vi "PrtSc + Crop image.vi"(11 "error in (no error)":errorcluster) -> (0 "error out":errorcluster, 3 "Image Dst Out":T1)   [LabVIEW 2011]
uses:
  <vilib>/vision/Image Controls.llb/IMAQ Image.ctl
  user32.dll
  <vilib>/vision/NI_Vision_Development_Module.lvlib
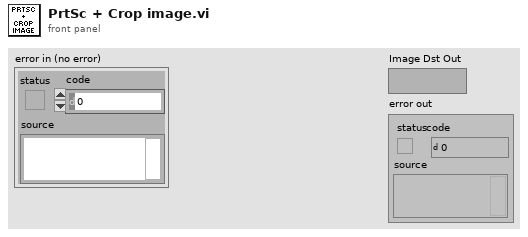
[diagram p1: front panel]
types:
  T1 = typedef "IMAQ Image.ctl" = refnum<image>
  T2 = typedef "Image Type" = u32
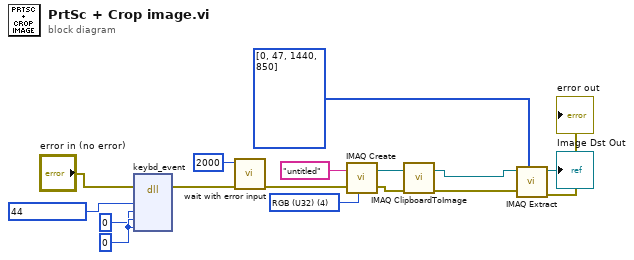
[diagram p0: block diagram]
diagram:
  w8 = T2 4 items=["Grayscale (U8)", "Grayscale (I16)", "Grayscale (SGL)", "Complex (CSG)", "RGB (U32)", "HSL (U32)", "RGB (U64)", "Grayscale (U16)"] ("Image Type")
  w16 = 0
  n1 = dll-call lib="user32.dll" fn="keybd_event"(error in="error in (no error)", u8 44 ("Virtual Key"), i8 0, w16, w16) -> (error out=w11:errorcluster)  [unwired: 7 in, 1 out]
  n2 = call "wait with error input.vi"("error in (no error)"=w11, "milliseconds to wait"=u32 2000) -> ("error out"=w10:errorcluster)  [unwired: 7 in, 2 out]
  n3 = call "IMAQ Create"("Image Name"="untitled", "Image Type"=w8, "error in (no error)"=w10) -> ("New Image"=w13:T1, "error out"=w4:errorcluster)  [unwired: 1 in, 1 out]
  n4 = call "IMAQ ClipboardToImage"("error in (no error)"=w4, "Image"=w13) -> ("error out"=w3:errorcluster, "Image Out"=w9:T1)  [unwired: 3 in, 2 out]
  n5 = call "IMAQ Extract"("Optional Rectangle"=i32[] [0, 47, 1440, 850], "error in (no error)"=w3, "Image Src"=w9) -> ("error out"=→"error out":errorcluster, "Image Dst Out"=→"Image Dst Out":T1)  [unwired: 7 in]
